vi "FG_Measure.vi"(0 "Peiker_Stepped Sweep Settings":T5={"Input Settings"={"IEPE min time to settle [s]"=0.0, "Responce Channel Settings"={"DSA response channel settings"={"coupling"=10045, "enable IEPE excitation"=FALSE, "IEPE current [mA]"=4.0}, "response channel info"={"sensor sensitivity"=1000.0, "engineering units"=1, "dB reference"=1.0, "custom label"="EU", "weighting filter"=0, "pregain"=0.0}, "AI response settings"={"response channel"="SOUNDACQ/ai1", "max value [V]"=10.0, "min value [V]"=-10.0, "terminal configuration"=-1}}, "Stimulus Channel Settings"={"AI stimulus settings"={"stimulus channel"="SOUNDACQ/ai0", "max value [V]"=10.0, "min value [V]"=-10.0, "terminal configuration"=-1}, "DSA stimulus channel settings"={"coupling"=10045, "enable IEPE excitation"=FALSE, "IEPE current [mA]"=4.0}, "stimulus channel info"={"sensor sensitivity"=1000.0, "engineering units"=1, "dB reference"=1.0, "custom label"="EU", "weighting filter"=0, "pregain"=0.0}}}, "Output Settings"={"AO source settings"={"excitation channel"="SOUNDACQ/ao0", "max value [V]"=10.0, "min value [V]"=-10.0, "terminal configuration"=-1}}} {"Output Settings"."AO source settings"."terminal configuration" items=["Default"=-1, "RSE"=10083, "Differential"=10106, "Pseudodifferential"=12529]; "Output Settings"."AO source settings"."min value [V]" format="%0.2f"; "Output Settings"."AO source settings"."max value [V]" format="%0.2f"; "Input Settings"."Stimulus Channel Settings"."stimulus channel info"."pregain" format="%.2f"; "Input Settings"."Stimulus Channel Settings"."stimulus channel info"."weighting filter" items=["Linear", "A-weighting", "B-weighting", "C-weighting", "ITU-R 468-4", "Dolby", "CCITT", "C-message", "Wb", "Wc", "Wd", "We", "Wf", "Wh", "Wj", "Wk", "Wm", "AES17 20 kHz lowpass", "AES17 40 kHz lowpass", "AES17 20 kHz highpass", "AES17 40 kHz highpass"]; "Input Settings"."Stimulus Channel Settings"."stimulus channel info"."dB reference" format="%^.1e"; "Input Settings"."Stimulus Channel Settings"."stimulus channel info"."engineering units" items=["custom..."=0, "V"=1, "A"=21, "C"=30, "pC"=31, "s"=32, "-"=29, "Pa"=2, "N"=20, "g"=3, "m/s^2"=4, "m/s"=5, "m"=6, "mm/s"=12, "mm"=13, "micron/s"=14, "micron"=15, "in/s^2"=7, "in/s"=8, "in"=9, "mil/s"=10, "mil"=11, "rad/s^2"=16, "rad/s"=17, "rad"=18, "deg/s^2"=26, "deg/s"=27, "deg"=28, "RPM"=22, "cycle/s^2"=23, "Hz"=24, "cycle"=25, "strain"=19]; "Input Settings"."Stimulus Channel Settings"."stimulus channel info"."sensor sensitivity" format="%#_5f"; "Input Settings"."Stimulus Channel Settings"."DSA stimulus channel settings"."IEPE current [mA]" format="%.1f"; "Input Settings"."Stimulus Channel Settings"."DSA stimulus channel settings"."coupling" items=["AC"=10045, "DC"=10050, "GND"=10066]; "Input Settings"."Stimulus Channel Settings"."AI stimulus settings"."terminal configuration" items=["Default"=-1, "RSE"=10083, "NRSE"=10078, "Differential"=10106, "Pseudodifferential"=12529]; "Input Settings"."Stimulus Channel Settings"."AI stimulus settings"."min value [V]" format="%.2f"; "Input Settings"."Stimulus Channel Settings"."AI stimulus settings"."max value [V]" format="%.2f"; "Input Settings"."Responce Channel Settings"."AI response settings"."terminal configuration" items=["Default"=-1, "RSE"=10083, "NRSE"=10078, "Differential"=10106, "Pseudodifferential"=12529]; "Input Settings"."Responce Channel Settings"."AI response settings"."min value [V]" format="%.2f"; "Input Settings"."Responce Channel Settings"."AI response settings"."max value [V]" format="%.2f"; "Input Settings"."Responce Channel Settings"."response channel info"."pregain" format="%.2f"; "Input Settings"."Responce Channel Settings"."response channel info"."weighting filter" items=["Linear", "A-weighting", "B-weighting", "C-weighting", "ITU-R 468-4", "Dolby", "CCITT", "C-message", "Wb", "Wc", "Wd", "We", "Wf", "Wh", "Wj", "Wk", "Wm", "AES17 20 kHz lowpass", "AES17 40 kHz lowpass", "AES17 20 kHz highpass", "AES17 40 kHz highpass"]; "Input Settings"."Responce Channel Settings"."response channel info"."dB reference" format="%^.1e"; "Input Settings"."Responce Channel Settings"."response channel info"."engineering units" items=["custom..."=0, "V"=1, "A"=21, "C"=30, "pC"=31, "s"=32, "-"=29, "Pa"=2, "N"=20, "g"=3, "m/s^2"=4, "m/s"=5, "m"=6, "mm/s"=12, "mm"=13, "micron/s"=14, "micron"=15, "in/s^2"=7, "in/s"=8, "in"=9, "mil/s"=10, "mil"=11, "rad/s^2"=16, "rad/s"=17, "rad"=18, "deg/s^2"=26, "deg/s"=27, "deg"=28, "RPM"=22, "cycle/s^2"=23, "Hz"=24, "cycle"=25, "strain"=19]; "Input Settings"."Responce Channel Settings"."response channel info"."sensor sensitivity" format="%#_5f"; "Input Settings"."Responce Channel Settings"."DSA response channel settings"."IEPE current [mA]" format="%.1f"; "Input Settings"."Responce Channel Settings"."DSA response channel settings"."coupling" items=["AC"=10045, "DC"=10050, "GND"=10066]; "Input Settings"."IEPE min time to settle [s]" format="%.1f"}, 1 "settling time":T11={"settle time [s]"=0.001, "settle cycles"=5} {"settle time [s]" format="%.2p"}, 2 "FrequencyList Output Level (dBSPL)":dbl=94.0, 5 "frequency list Input":T4(array[cluster])=[{"frequency [Hz]"=200.0, "amplitude [V]"=0.5}, {"frequency [Hz]"=224.0, "amplitude [V]"=0.5}, {"frequency [Hz]"=250.0, "amplitude [V]"=0.5}, {"frequency [Hz]"=280.0, "amplitude [V]"=0.5}, {"frequency [Hz]"=315.0, "amplitude [V]"=0.5}, {"frequency [Hz]"=355.0, "amplitude [V]"=0.5}, {"frequency [Hz]"=400.0, "amplitude [V]"=0.5}, {"frequency [Hz]"=450.0, "amplitude [V]"=0.5}, {"frequency [Hz]"=500.0, "amplitude [V]"=0.5}, {"frequency [Hz]"=560.0, "amplitude [V]"=0.5}, {"frequency [Hz]"=630.0, "amplitude [V]"=0.5}, {"frequency [Hz]"=710.0, "amplitude [V]"=0.5}, {"frequency [Hz]"=800.0, "amplitude [V]"=0.5}, {"frequency [Hz]"=900.0, "amplitude [V]"=0.5}, {"frequency [Hz]"=1000.0, "amplitude [V]"=0.5}, {"frequency [Hz]"=1120.0, "amplitude [V]"=0.5}, {"frequency [Hz]"=1250.0, "amplitude [V]"=0.5}, {"frequency [Hz]"=1400.0, "amplitude [V]"=0.5}, {"frequency [Hz]"=1600.0, "amplitude [V]"=0.5}, {"frequency [Hz]"=1800.0, "amplitude [V]"=0.5}, {"frequency [Hz]"=2000.0, "amplitude [V]"=0.5}, {"frequency [Hz]"=2240.0, "amplitude [V]"=0.5}, {"frequency [Hz]"=2500.0, "amplitude [V]"=0.5}, {"frequency [Hz]"=2800.0, "amplitude [V]"=0.5}, {"frequency [Hz]"=3150.0, "amplitude [V]"=0.5}, {"frequency [Hz]"=3550.0, "amplitude [V]"=0.5}, {"frequency [Hz]"=4000.0, "amplitude [V]"=0.5}, {"frequency [Hz]"=4500.0, "amplitude [V]"=0.5}, {"frequency [Hz]"=5000.0, "amplitude [V]"=0.5}, {"frequency [Hz]"=5600.0, "amplitude [V]"=0.5}, {"frequency [Hz]"=6300.0, "amplitude [V]"=0.5}, {"frequency [Hz]"=7100.0, "amplitude [V]"=0.5}, {"frequency [Hz]"=8000.0, "amplitude [V]"=0.5}] {"amplitude [V]" format="%.6f"; "frequency [Hz]" format="%.2f"}, 9 "true=mehrfach Messen":bool, 11 "error in (no error)":errorcluster, 12 "FrequencyList Input Level (dBSPL)":dbl=94.0, 13 "integration time":T10={"integration time [s]"=0.001, "integration cycles"=5} {"integration cycles" min=2; "integration time [s]" format="%.2p"}) -> (3 "Fundamental-Response":T3(graph), 4 "THD-Response":cluster{"frequency":dbl[], "THD":dbl[]}(graph), 6 "Harmonics-Response":cluster{"frequency":dbl[], "distortion":dbl[]}[](graph), 10 "Response Level":cluster{"frequency":dbl[], "magnitude":dbl[]}(graph), 14 "Stimulus Level":cluster{"frequency":dbl[], "magnitude":dbl[]}(graph), 15 "error out":errorcluster={"status"=FALSE, "code"=0, "source"="\r\n"})   [LabVIEW 2018]
doc: "Das VI dient dem Messen eines Frequenzgangs. \nDieser kann verwendet werden um den Speaker abzugleichen.\nEin abweichender Pegel darf erst angegeben werden, wenn ein Speakerabgleich auf 94 dBSpl erfolgt ist.\n\nDie 94dB Spannungswerte werden dann auf den gewünschten Pegel umgerechnet."
uses:
  Peiker_Stepped Sweep Settings.ctl
  <vilib>/addons/_NISVFA/_Shared subVIs/Controls/svc_DSA Channel Settings.ctl
  <vilib>/addons/_NISVFA/_Shared subVIs/Controls/svc_Channel Info.ctl
  <vilib>/addons/_NISVFA/_Shared subVIs/Controls/svc_Engineering Units Text Ring.ctl
  <vilib>/addons/_NISVFA/_Shared subVIs/Controls/svc_Weighting Filter Text Ring.ctl
  <vilib>/addons/_NISVFA/_Baseband FFT/SVFA Power Spectrum (N Ch).vi
  <vilib>/addons/Sound and Vibration/svt_Swept Sine/SoundVib_SweptSine.lvlib
panel:
  out "Counter":i32
  out "Waveform Graph 4":waveform(dbl)[](graph)
  in  "Tab Control":T1(tab)
  out "Waveform Graph 2":waveform(dbl)[](graph)
  in  "Messkurve":dbl min=0.0 max=28.0
  out "Block Duration":waveform(dbl)[](graph)
  in  "stop":bool
  in  "Enable this Diagramm":bool
  out "Waveform Graph 3":cluster{"f0":dbl, "df":dbl, "magnitude":dbl[]}[](graph)
  out "Fundamental-Response dB berechnet":T2(graph) caption="Fundamental-Response dB berechnet aus THD-Modul"
  out "THD":cluster{"frequency":dbl[], "THD":dbl[]}={"frequency"=[103.0], "THD"=[0.2630754420190896]} {"THD" format="%.2f"; "frequency" format="%.2f"}
  out "Waveform Graph":cluster{"f0":dbl, "df":dbl, "magnitude":dbl[]}[](graph)
  out "FrequencyList Output Level":T4(graph)
  in  "Anzahl der Messungen bei einer Frequenz":i32=10
  in  "block duration [ms]":dbl=100.0
  in  "sample rate [Hz]":dbl=100000.0
  out "status":T12 {"% complete" format="%.2f"; "current processed frequency" format="%.2f"; "current source frequency" format="%.2f"; "elapsed time [s]" format="%.2f"}
  # "200_Hz\n224_Hz\n250_Hz\n280_Hz\n315_Hz\n355_Hz\n400_Hz\n450_Hz\n500_Hz\n560_Hz\n630_Hz\n710_Hz\n800_Hz\n900_Hz\n1000_Hz\n1120_Hz\n1250_Hz\n1400_Hz\n1600_Hz\n1800_Hz\n2000_Hz\n2240_Hz\n2500_Hz\n2800_Hz\n3150_Hz\n3550_Hz\n4000_Hz\n4500_Hz\n5000_Hz\n5600_Hz\n6300_Hz\n7100_Hz\n8000_Hz"
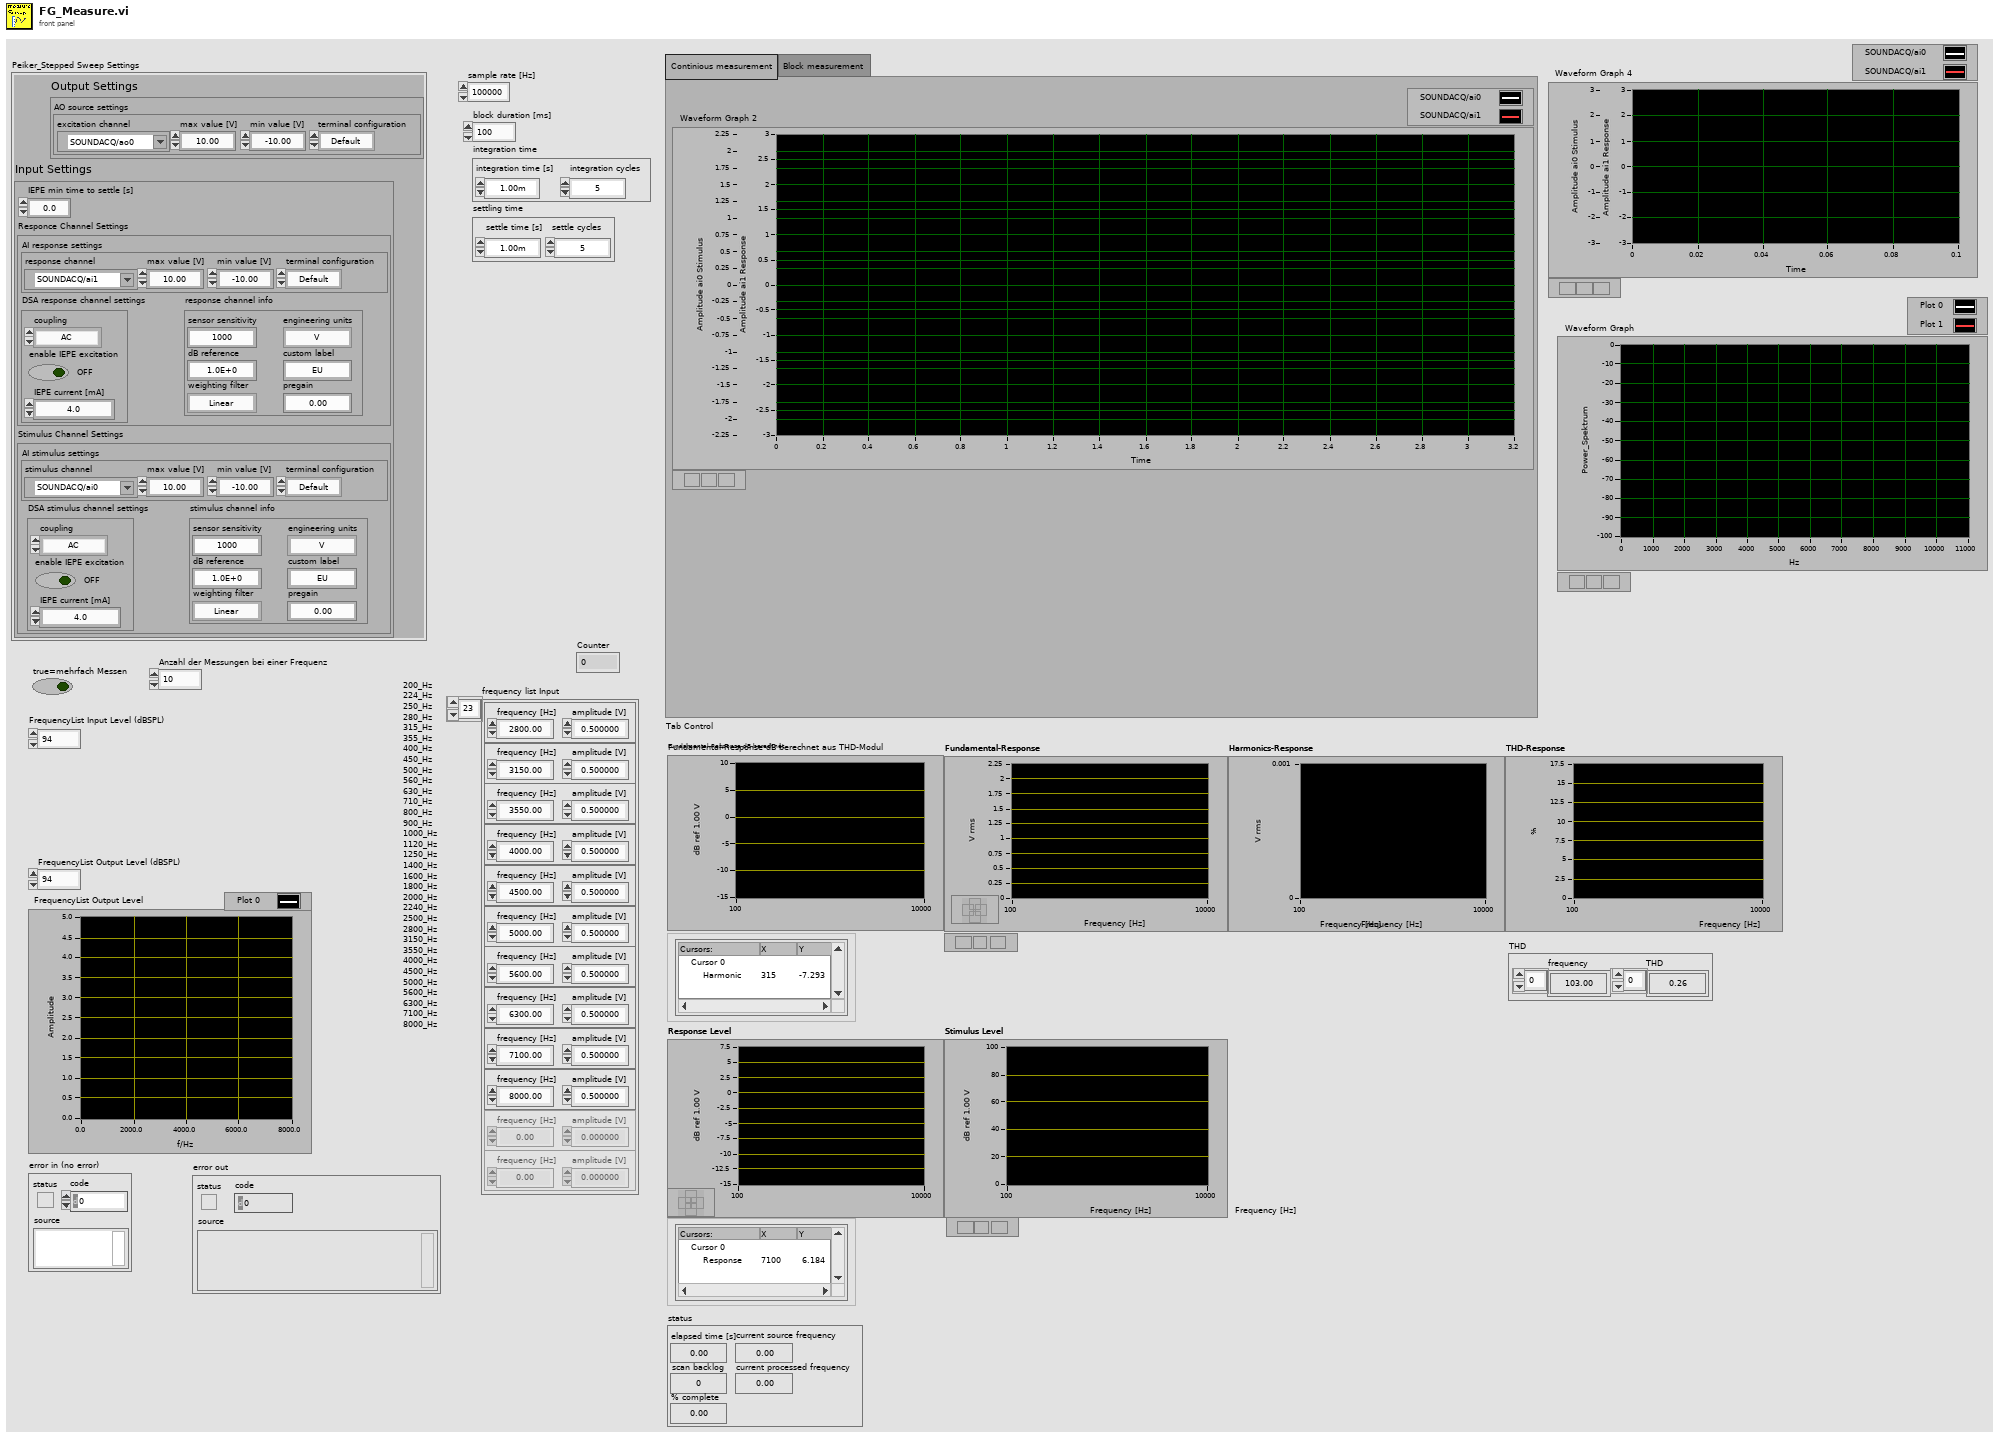
[diagram p1: front panel]
types:
  T1 = enum32{"Continious measurement", "Block measurement"}
  T2 = cluster{"frequency [Hz]":dbl[], "amplitude":dbl[]}[]
  T3 = cluster{"frequency [Hz]":dbl[], "amplitude":dbl[]}
  T4 = cluster{"frequency [Hz]":dbl, "amplitude [V]":dbl}[]
  T5 = typedef "Peiker_Stepped Sweep Settings.ctl" = cluster{"Input Settings":cluster{"IEPE min time to settle [s]":dbl, "Responce Channel Settings":cluster{"DSA response channel settings":T6, "response channel info":T7, "AI response settings":cluster{"response channel":tag, "max value [V]":dbl, "min value [V]":dbl, "terminal configuration":i32}}, "Stimulus Channel Settings":cluster{"AI stimulus settings":cluster{"stimulus channel":tag, "max value [V]":dbl, "min value [V]":dbl, "terminal configuration":i32}, "DSA stimulus channel settings":T6, "stimulus channel info":T7}}, "Output Settings":cluster{"AO source settings":cluster{"excitation channel":tag, "max value [V]":dbl, "min value [V]":dbl, "terminal configuration":i32}}}
  T6 = typedef "svc_DSA Channel Settings.ctl" = cluster{"coupling":i32, "enable IEPE excitation":bool, "IEPE current [mA]":dbl}
  T7 = typedef "svc_Channel Info.ctl" = cluster{"sensor sensitivity":dbl, "engineering units":T8, "dB reference":dbl, "custom label":string, "weighting filter":T9, "pregain":dbl}
  T8 = typedef "svc_Engineering Units Text Ring.ctl" = u16
  T9 = typedef "svc_Weighting Filter Text Ring.ctl" = u16
  T10 = cluster{"integration time [s]":dbl, "integration cycles":i32}
  T11 = cluster{"settle time [s]":dbl, "settle cycles":i32}
  T12 = cluster{"elapsed time [s]":dbl, "scan backlog":u32, "current source frequency":dbl, "current processed frequency":dbl, "% complete":dbl}
  T13 = cluster{"excitation channel":tag, "max value [V]":dbl, "min value [V]":dbl, "terminal configuration":i32}
  T14 = cluster{"stimulus channel":tag, "max value [V]":dbl, "min value [V]":dbl, "terminal configuration":i32}
  T15 = cluster{"response channel":tag, "max value [V]":dbl, "min value [V]":dbl, "terminal configuration":i32}
  T16 = typedef "SoundVib_SweptSine.lvlib/sv_Swept Sine Task.ctl" = cluster{"source settings":cluster{"AO task name":refnum<k21>, "source":cluster{"AO physical channel":tag}[]}, "stimulus settings":cluster{"stimulus task name":refnum<k21>, "stimulus":cluster{"stimulus physical channel":tag, "channel info":T7}[]}, "response(s) settings":cluster{"response task name":refnum<k21>, "response":cluster{"response physical channel":tag, "channel info":T7}[]}, "measurement settings":cluster{"AI sampling frequency":dbl, "AO sampling frequency":dbl, "AI block size":i32, "AO block Size":i32, "block duration [ms]":dbl, "number of AI channels":i32, "device propagation delay [samples]":dbl, "total propagation time [samples]":dbl, "DUT propagation time [ms]":dbl}, "linlog":enum16{"linear", "log"}, "repeat":enum16{"off", "on"}, "frequency list":dbl[], "amplitude list":dbl[], "settling time":cluster{"settle time":dbl, "settle cycles":i32}, "integration time":cluster{"integration time":dbl, "integration cycles":i32}, "frequencies indices":cluster{"AI freq index":i32, "AO freq index":i32}, "read marks":cluster{"write index":u32, "read index":u32, "freq start index":u32, "freq stop index":u32, "# extracted":u32, "buffer type":enum16{"Invalid buffer", "Intermediate buffer", "Final buffer"}, "read/write indices":cluster{"settle time index":u32, "integration time index":u32}[], "AO index":i32, "AI index":i32, "settled":bool, "integration done":bool}, "harmonic settings":cluster{"maximum THD harmonic":u32, "harmonic mapping":u32[], "units":cluster{"THD unit":enum16{"dB", "%"}, "nth harmonic unit":enum16{"dB", "%"}, "SINAD unit":enum16{"dB", "%"}, "THD+N unit":enum16{"dB", "%"}}}, "auto resolution settings":cluster{"auto max step":i32, "slow threshold db":dbl, "fast threshold db":dbl}, "auto level settings":cluster{"auto level enable":bool, "auto level channel":u8, "ideal ref":sgl, "max level":sgl, "ref upper deviation db":sgl, "ref lower deviation db":sgl}, "offset":dbl, "ramping rate":dbl, "phase":dbl, "initialize":bool}
  T17 = enum16{"EU rms", "EU peak", "EU peak-peak", "dB ref fund"}
  T18 = cluster{"THD units":enum16{"dB", "linear ratio", "%"}, "harmonic component amplitude units":enum16{"EU rms", "EU peak", "EU peak-peak", "dB ref fund"}, "fundamental amplitude units":enum16{"EU rms", "EU peak", "EU peak-peak"}}
  T19 = typedef "SoundVib_SweptSine.lvlib/sv_Swept Sine Measurements.ctl" = cluster{"RMS stimulus":dbl[], "RMS response":dbl[], "Re [stimulus]":dbl[], "Im [stimulus]":dbl[], "Re [response]":dbl[], "Im [response]":dbl[], "THD":dbl[], "Harm[]":dbl[][], "scaled response magnitude":dbl[]}
  T20 = cluster{"THD unit label":string, "harmonic component amplitudes unit label":string, "fundamental amplitude unit label":string}
  T21 = cluster{"response physical channel":tag, "channel info":T7}[]
  T22 = cluster{"response physical channel":tag, "channel info":T7}
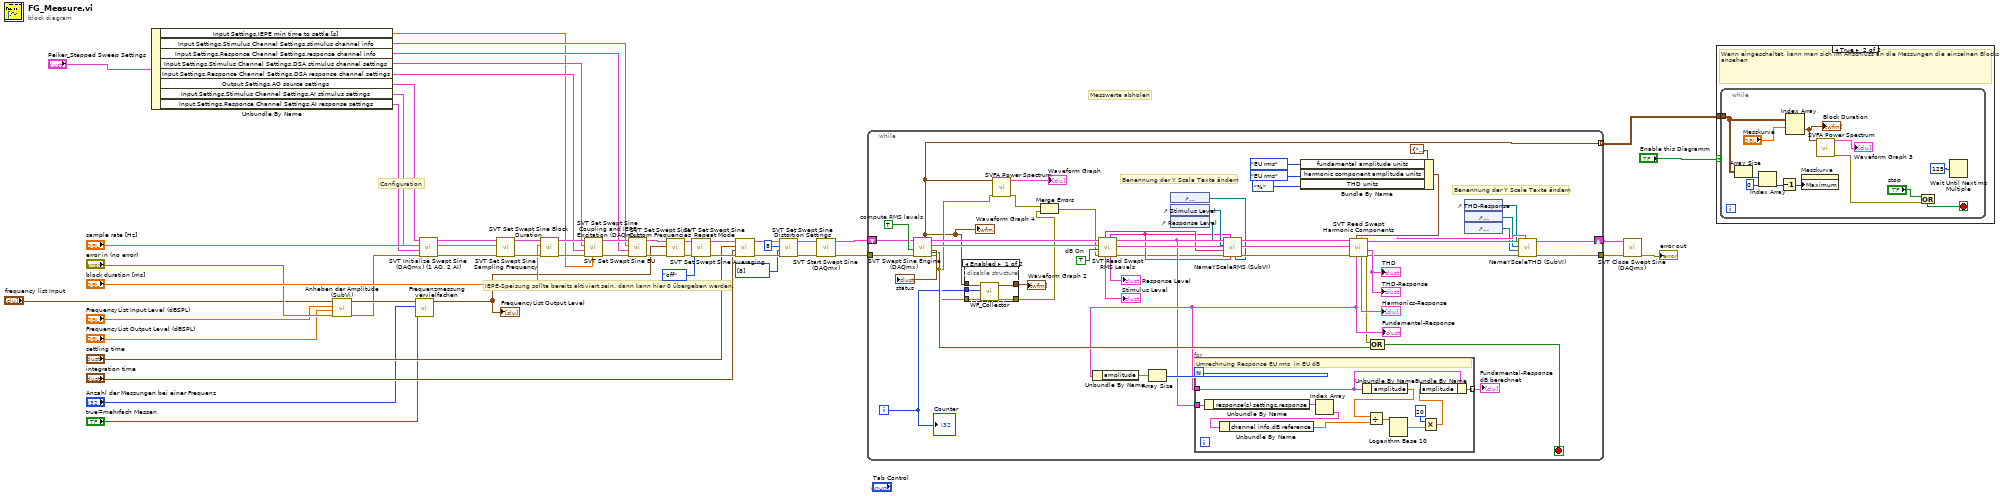
[diagram p0: block diagram]
diagram:
  # "IEPE-Speisung sollte bereits aktiviert sein. dann kann hier 0 übergeben werden."
  # "Messwerte abholen"
  # "Configuration"
  n1 = Unbundle By Name("Peiker_Stepped Sweep Settings") -> ("Input Settings.IEPE min time to settle [s]"=w21:dbl, "Input Settings.Stimulus Channel Settings.stimulus channel info"=w24:T7, "Input Settings.Responce Channel Settings.response channel info"=w25:T7, "Input Settings.Stimulus Channel Settings.DSA stimulus channel settings"=w26:T6, "Input Settings.Responce Channel Settings.DSA response channel settings"=w27:T6, "Output Settings.AO source settings"=w33:T13, "Input Settings.Stimulus Channel Settings.AI stimulus settings"=w3:T14, "Input Settings.Responce Channel Settings.AI response settings"=w2:T15)
  n2 = call "Anheben der Amplitude (SubVi).vi"("error In"="error in (no error)", "FrequencyList Output Level (calc)"="FrequencyList Output Level (dBSPL)", "FrequencyList Input Level"="FrequencyList Input Level (dBSPL)", "custom frequency list Input"="frequency list Input") -> ("error Out"=w14:errorcluster, "custom frequency list Output"=w17:T4)  [unwired: 5 in, 1 out]
  n3 = call "Frequenzmessung vervielfachen.vi"("true=mehrfach Messen"="true=mehrfach Messen", "Anzahl der Messungen bei einer Frequenz"="Anzahl der Messungen bei einer Frequenz", "Eingang"=w17) -> ("Ausgang"=w18:T4)  [unwired: 8 in]
  "FrequencyList Output Level" <- w18
  n4 = call <vilib>:"SVT Initialize Swept Sine (DAQmx) (1 AO, 2 AI).vi"("error in (no error)"=w14, "AI response settings"=w2, "AI stimulus settings"=w3, "AO source settings"=w33) -> ("error out"=w9:errorcluster, "swept sine task out"=w8:T16)  [unwired: 6 in]
  n5 = call <vilib>:"SVT Set Swept Sine Sampling Frequency.vi"("error in (no error)"=w9, "sampling frequency\n[samples/s]"="sample rate [Hz]", "swept sine task in"=w8) -> ("error out"=w38:errorcluster, "swept sine task out"=w39:T16)  [unwired: 7 in]
  n6 = call <vilib>:"SVT Set Swept Sine Block Duration.vi"("error in (no error)"=w38, "block duration [ms]"="block duration [ms]", "swept sine task in"=w39) -> ("error out"=w50:errorcluster, "swept sine task out"=w49:T16)  [unwired: 7 in]
  n7 = call <vilib>:"SVT Set Swept Sine Coupling and IEPE Excitation (DAQmx).vi"("time to settle [s]"=w21, "error in (no error)"=w50, "DSA response channel settings"=w27, "DSA stimulus channel settings"=w26, "swept sine task in"=w49) -> ("error out"=w47:errorcluster, "swept sine task out"=w48:T16)  [unwired: 5 in]
  n8 = call <vilib>:"SVT Set Swept Sine EU.vi"("error in (no error)"=w47, "response channel info"=w25, "stimulus channel info"=w24, "swept sine task in"=w48) -> ("error out"=w46:errorcluster, "swept sine task out"=w45:T16)  [unwired: 6 in]
  n9 = call <vilib>:"SVT Set Swept Sine Custom Frequencies.vi"("error in (no error)"=w46, "custom frequency list"=w18, "swept sine task in"=w45) -> ("error out"=w36:errorcluster, "swept sine task out"=w37:T16)  [unwired: 7 in]
  n10 = call <vilib>:"SVT Set Swept Sine Repeat Mode.vi"("error in (no error)"=w36, "repeat"=enum16{"off", "on"}."off", "swept sine task in"=w37) -> ("error out"=w44:errorcluster, "swept sine task out"=w43:T16)  [unwired: 7 in]
  n11 = call <vilib>:"SVT Set Swept Sine Averaging.vi"("error in (no error)"=w44, "integration time"="integration time", "settling time"="settling time", "swept sine task in"=w43) -> ("error out"=w41:errorcluster, "swept sine task out"=w42:T16)  [unwired: 6 in]
  n12 = call <vilib>:"SVT Set Swept Sine Distortion Settings.vi"("error in (no error)"=w41, "harmonics to visualize"=u32[] [8], "maximum harmonic"=u32 8, "swept sine task in"=w42) -> ("error out"=w6:errorcluster, "swept sine task out"=w7:T16)  [unwired: 6 in]
  n13 = call <vilib>:"SVT Start Swept Sine (DAQmx).vi"("error in (no error)"=w6, "swept sine task in"=w7) -> ("error out"=w5:errorcluster, "swept sine task out"=w4:T16)  [unwired: 8 in]
  n14 = while {
    tunnel: w5 -> [w90]
    tunnel: [w59] -> w40
    shift-right: [w87] -> w16
    shift-left: w4 -> [w86]
    tunnel: [w51] -> w11 mode=indexing
    i -> [w56]
    stop <- w89 stop-if-true
    w93 = TRUE  # dB On
    w95 = TRUE  # compute RMS levels
    # "Benennung der Y Scale Texte ändern"
    # "Benennung der Y Scale Texte ändern"
    n15 = call <vilib>:"SVT Swept Sine Engine (DAQmx).vi"("error in (no error)"=w90, "compute RMS levels (F)"=w95, "swept sine task in"=w86) -> ("error out"=w55:errorcluster, "status"=→"status":T12, "swept sine measurements"=w75:T19, "swept sine task out"=w94:T16, "sweep done"=w88:bool, "waveform data [V]"=w51:waveform(dbl)[])  [unwired: 3 in]
    "Waveform Graph 4" <- w51
    n16 = disable-structure shown="Enabled" {
      disable-tunnel: w51 -> [w101 w102]
      disable-tunnel: w56 -> [w100 _]
      disable-tunnel: w55 -> [w99 w103]
      disable-tunnel: [w98 w103] -> w53
      disable-tunnel: [w97 w102] -> w57
      frame Enabled {
        n17 = call "WF_Collector.vi"("error in (no error)"=w99, "LoopCounter"=w100, "waveform data ClusterIn"=w101) -> ("error out"=w98:errorcluster, "waveform data ClusterOut"=w97:waveform(dbl)[])  [unwired: 7 in]
      }
      frame Disabled {
      }
    }
    "Waveform Graph 2" <- w57
    n18 = call-poly <vilib>:"SVFA Power Spectrum.vi"("scaled signals [EU]"=w51, "error in (no error)"=w55) -> ("power spectra [dB EU]"=→"Waveform Graph":cluster{"f0":dbl, "df":dbl, "magnitude":dbl[]}[], "error out"=w54:errorcluster)  [unwired: 12 in, 4 out]
    n19 = Merge Errors(w54, w53) -> (w52:errorcluster)
    n20 = call <vilib>:"SVT Read Swept RMS Levels.vi"("error in (no error)"=w52, "dB On (T)"=w93, "swept sine measurements"=w75, "swept sine task in"=w94) -> ("error out"=w58:errorcluster, "dup swept sine measurements"=w72:T19, "swept sine task out"=w71:T16, "RMS level (response)"=→"Response Level":cluster{"frequency":dbl[], "magnitude":dbl[]}, "response unit label"=w61:string, "RMS level (stimulus)"=→"Stimulus Level":cluster{"frequency":dbl[], "magnitude":dbl[]}, "stimulus unit label"=w64:string)  [unwired: 1 in]
    n21 = control-ref of="Fundamental-Response dB berechnet"() -> (w60:refnum<vi>)
    n22 = control-ref of="Stimulus Level"() -> (w62:refnum<vi>)
    n23 = control-ref of="Response Level"() -> (w63:refnum<vi>)
    n24 = call "NameYScaleRMS (SubVI).vi"("XYGraph in 2"=w60, "response unit label 2"=w61, "response unit label"=w61, "error in (no error)"=w58, "stimulus unit label"=w64, "XYGraph Refnum in"=w62, "XYGraph in"=w63) -> ("error out"=w65:errorcluster)  [unwired: 4 in]
    n25 = Bundle By Name(cluster=T18 {"THD units"=enum."dB", "harmonic component amplitude units"=enum."EU rms", "fundamental amplitude units"=enum."EU rms"} ("output cluster"), "fundamental amplitude units"=enum16{"EU rms", "EU peak", "EU peak-peak"}."EU rms", "harmonic component amplitude units"=T17."EU rms", "THD units"=enum16{"dB", "linear ratio", "%"}."%") -> (w80:T18)
    n26 = call <vilib>:"SVT Read Swept Harmonic Components.vi"("desired units"=w80, "error in (no error)"=w65, "swept sine measurements"=w72, "swept sine task in"=w71) -> ("error out"=w70:errorcluster, "THD"=→"THD-Response" →"THD":cluster{"frequency":dbl[], "THD":dbl[]}, "swept sine task out"=w87:T16, "harmonic components"=→"Harmonics-Response":cluster{"frequency":dbl[], "distortion":dbl[]}[], "unit labels"=w69:T20, "fundamental amplitude"=w76:T3)  [unwired: 1 in, 1 out]
    "Fundamental-Response" <- w76
    n27 = Unbundle By Name(w76) -> ("amplitude"=w83:dbl[])
    n28 = Array Size(array=w83) -> (size(s)=w82:i32)
    n29 = for {
      N: w82 -> [_]
      tunnel: w76 -> [w110]
      tunnel: [w108] -> w84 mode=indexing
      tunnel: w71 -> [w106]
      # "Umrechnung Response EU rms  in EU dB"
      n30 = Unbundle By Name(w106) -> ("response(s) settings.response"=w105:T21)
      n31 = Index Array(array=w105) -> (element=w107:T22)  [unwired: 1 in]
      n32 = Unbundle By Name(w107) -> ("channel info.dB reference"=w104:dbl)
      n33 = Unbundle By Name(w110) -> ("amplitude"=w113:dbl[])
      n34 = Divide(x=w113, y=w104) -> (x/y=w114:dbl[])
      n35 = Logarithm Base 10(1:w114) -> (0:w111:dbl[])
      n36 = Multiply(x=20, y=w111) -> (x*y=w109:dbl[])
      n37 = Bundle By Name(cluster=w110, "amplitude"=w109) -> (w108:T3)
    }
    "Fundamental-Response dB berechnet" <- w84
    n38 = Compound Arithmetic op=OR(w70, w88) -> (w89:bool)
    n39 = control-ref of="THD-Response"() -> (w68:refnum<vi>)
    n40 = control-ref of="Harmonics-Response"() -> (w67:refnum<vi>)
    n41 = control-ref of="Fundamental-Response"() -> (w66:refnum<vi>)
    n42 = call "NameYScaleTHD (SubVI).vi"("unit labels"=w69, "error in (no error)"=w70, "XYGraph Refnum 3"=w66, "XYGraph Refnum in"=w67, "XYGraph in"=w68) -> ("error out"=w59:errorcluster)  [unwired: 6 in]
    "Counter" <- w56
  }
  n43 = call <vilib>:"SVT Close Swept Sine (DAQmx).vi"("error in (no error)"=w40, "swept sine task in"=w16) -> ("error out"=→"error out":errorcluster)  [unwired: 9 in]
  n44 = case shown="True" "Enable this Diagramm" {
    tunnel: w11 -> [_ w115]
    frame False {
    }
    frame True {
      # "Wenn eingeschaltet, kann man sich im Anschluss an die Messungen die einzelnen Blocks ansehen"
      n45 = while {
        tunnel: w115 -> [w118]
        stop <- w117 stop-if-true
        n46 = Array Size(array=w118) -> (size(s)=w122:i32[])
        n47 = Index Array(array=w122, index=0) -> (element=w120:i32)
        n48 = Decrement(x=w120) -> (x-1=w119:i32)
        n49 = Index Array(array=w118, index (row)="Messkurve") -> (element=w124:waveform(dbl)[])  [unwired: 1 in]
        "Block Duration" <- w124
        n50 = property on="Messkurve" class="DigNum (strict)"("Maximum"=w119) -> ()  [unwired: 2 in, 2 out]
        n51 = call-poly <vilib>:"SVFA Power Spectrum.vi"("scaled signals [EU]"=w124) -> ("power spectra [dB EU]"=→"Waveform Graph 3":cluster{"f0":dbl, "df":dbl, "magnitude":dbl[]}[], "error out"=w116:errorcluster)  [unwired: 13 in, 4 out]
        n52 = Or(x="stop", y=w116) -> (x .or. y?=w117:bool)
        n53 = Wait Until Next ms Multiple(millisecond multiple=u32 125) -> ()  [unwired: 1 out]
      }
    }
  }
